vi "Breakdown ROI to miniscans.vi"(11 "ROI Attributes":T1[](array[typedef]) {"ROI group ID" format="%#_6f"; "Laser Power (%)" format="%#_6f"; "Zoom" format="%#_6f"; "Frame Size" format="%#_6f"; "Number of lines" format="%#_6f"; "Composite ID" format="%#_6f"; "Angle (deg)" format="%#_6f"; "ROI Time (ns)" format="%#_6f"; "ROI ID" format="%#_6f"; "Pixels in ROI" format="%#_6f"; "ROI index" format="%#_6f"; "Z stop" format="%#_6f"; "Y stop" format="%#_6f"; "X stop" format="%#_6f"; "Z start" format="%#_6f"; "X start" format="%#_6f"; "Y start" format="%#_6f"}) -> (1 "Laser(V)":dbl[](array[numeric]), 3 "ROI Attributes (broken down to miniscans)":T1[](array[typedef]) {"ROI group ID" format="%#_6f"; "Laser Power (%)" format="%#_6f"; "Zoom" format="%#_6f"; "Frame Size" format="%#_6f"; "Number of lines" format="%#_6f"; "Composite ID" format="%#_6f"; "Angle (deg)" format="%#_6f"; "ROI Time (ns)" format="%#_6f"; "ROI ID" format="%#_6f"; "Pixels in ROI" format="%#_6f"; "ROI index" format="%#_6f"; "Z stop" format="%#_6f"; "Y stop" format="%#_6f"; "X stop" format="%#_6f"; "Z start" format="%#_6f"; "X start" format="%#_6f"; "Y start" format="%#_6f"})   [LabVIEW 2017]
uses:
  User Interface/Visualisation/Functional Imaging Viewer/Typedefs/ROI parameters data type.ctl
  Global Variables/General Globals.vi
panel:
  out "Output size":i32
  out "Input size":i32
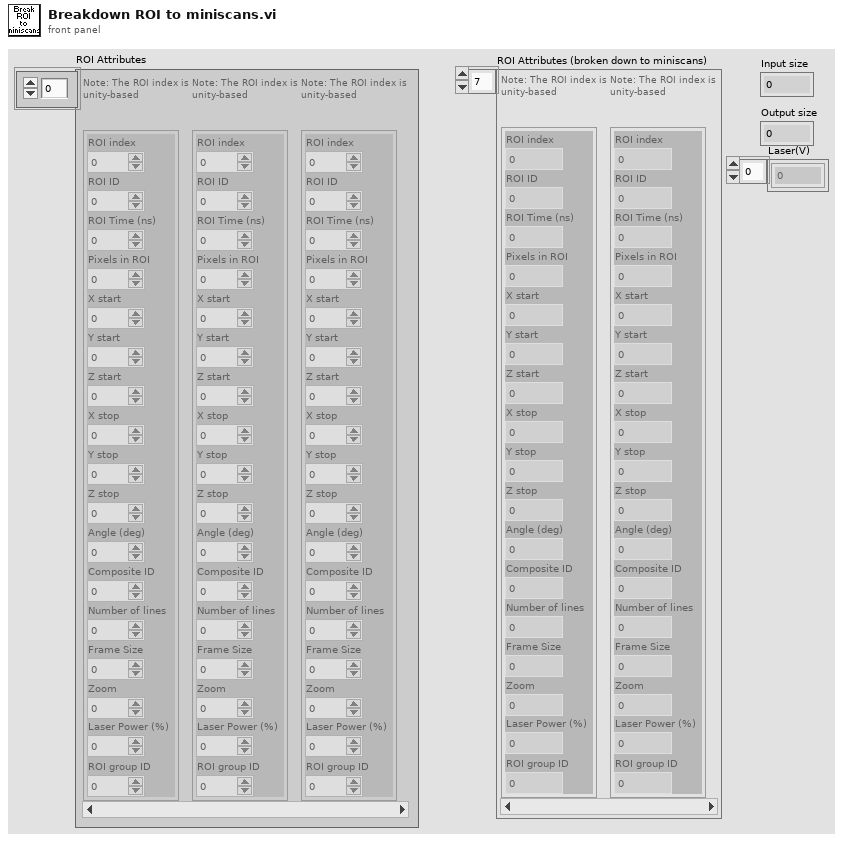
[diagram p1: front panel]
types:
  T1 = typedef "ROI parameters data type.ctl" = cluster{"ROI index":dbl, "ROI ID":dbl, "ROI Time (ns)":dbl, "Pixels in ROI":dbl, "X start":dbl, "Y start":dbl, "Z start":dbl, "X stop":dbl, "Y stop":dbl, "Z stop":dbl, "Angle (deg)":dbl, "Composite ID":dbl, "Number of lines":dbl, "Frame Size":dbl, "Zoom":dbl, "Laser Power (%)":dbl, "ROI group ID":dbl}
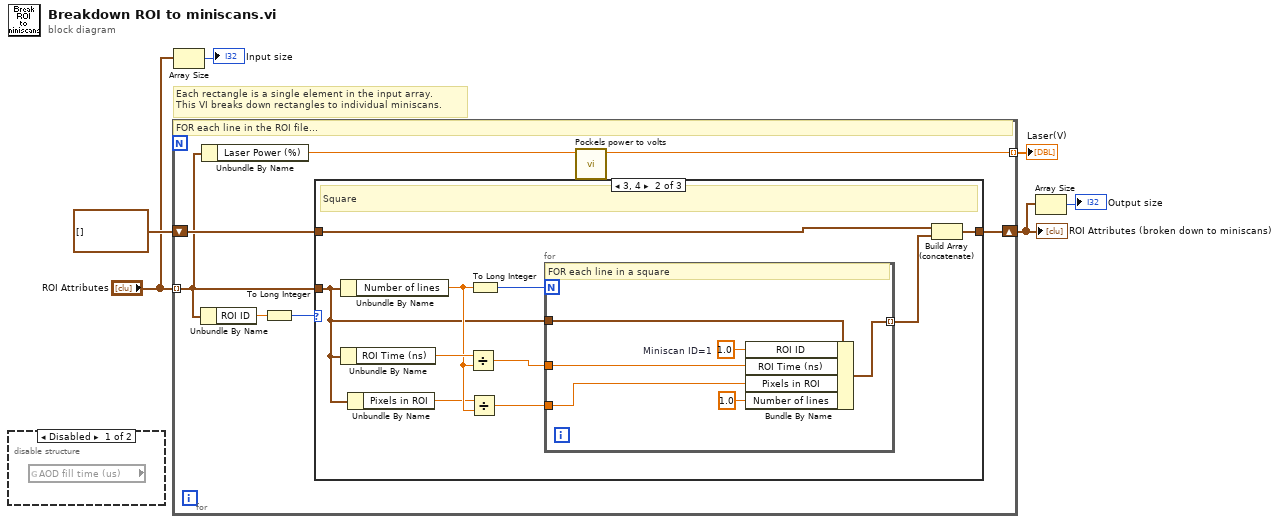
[diagram p0: block diagram]
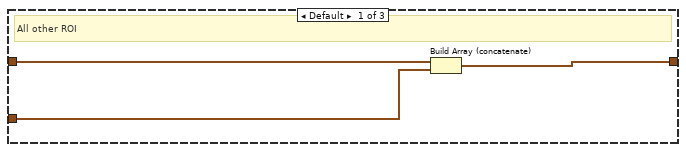
[diagram p3: hidden frame]
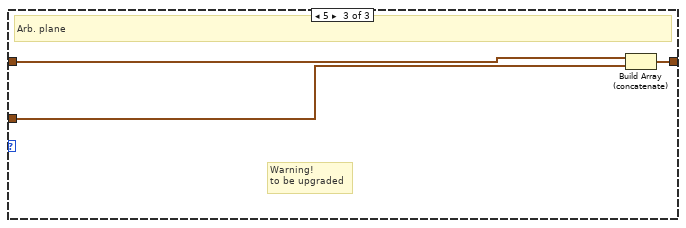
[diagram p4: hidden frame]
diagram:
  # "Each rectangle is a single element in the input array.\nThis VI breaks down rectangles to individual miniscans."
  n1 = disable-structure shown="Disabled" {
    frame Disabled {
      n2 = global read "General Globals.vi" "AOD fill time (us)"() -> ()  [unwired: 1 out]
    }
    frame Enabled {
    }
  }
  n3 = for {
    tunnel: "ROI Attributes" -> [w9] mode=indexing
    shift-right: [w10] -> w2
    shift-left: T1[] [] ("ROI Coordinates (broken down to miniscans)") -> [w11]
    tunnel: [w7] -> w1 mode=indexing
    # "FOR each line in the ROI file..."
    n4 = Unbundle By Name(w9) -> ("ROI ID"=w13:dbl)
    n5 = Unbundle By Name(w9) -> ("Laser Power (%)"=w8:dbl)
    n6 = To Long Integer(number=w13) -> (32bit integer=w12:i32)
    n7 = case shown="3, 4" w12 {
      tunnel: w9 -> [w15 w20 w33]
      tunnel: [w14 w25 w35] -> w10
      tunnel: w11 -> [w16 w24 w34]
      frame Default {
        # "All other ROI"
        n8 = Build Array (concatenate)(w16, w15) -> (w14:T1[])
      }
      frame 3, 4 {
        # "Square"
        n9 = Unbundle By Name(w20) -> ("Number of lines"=w21:dbl)
        n10 = Unbundle By Name(w20) -> ("ROI Time (ns)"=w23:dbl)
        n11 = Unbundle By Name(w20) -> ("Pixels in ROI"=w19:dbl)
        n12 = Divide(x=w23, y=w21) -> (x/y=w17:dbl)
        n13 = Divide(x=w19, y=w21) -> (x/y=w18:dbl)
        n14 = To Long Integer(number=w21) -> (32bit integer=w22:i32)
        n15 = for {
          N: w22 -> [_]
          tunnel: w20 -> [w32]
          tunnel: [w31] -> w26 mode=indexing
          tunnel: w17 -> [w29]
          tunnel: w18 -> [w28]
          w30 = 1.0  # Miniscan ID=1
          # "FOR each line in a square"
          n16 = Bundle By Name(cluster=w32, "ROI ID"=w30, "ROI Time (ns)"=w29, "Pixels in ROI"=w28, "Number of lines"=1.0) -> (w31:T1)
        }
        n17 = Build Array (concatenate)(w24, w26) -> (w25:T1[])
      }
      frame 5 {
        # "Warning!\nto be upgraded"
        # "Arb. plane"
        n18 = Build Array (concatenate)(w34, w33) -> (w35:T1[])
      }
    }
    n19 = call "Pockels power to volts.vi"("Pockels power (%)"=w8) -> ("Pockels control voltage (V)"=w7:dbl)  [unwired: 8 in, 2 out]
  }
  "ROI Attributes (broken down to miniscans)" <- w2
  "Laser(V)" <- w1
  n20 = Array Size(array="ROI Attributes") -> (size(s)=→"Input size":i32)
  n21 = Array Size(array=w2) -> (size(s)=→"Output size":i32)
